vi "Ball Intake System.vi"(10 "Outtake":bool, 11 "Intake":bool) -> ()   [LabVIEW 2018]
panel:
  in  "Scaling factor":dbl=0.5
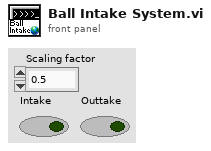
[diagram p1: front panel]
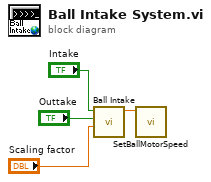
[diagram p0: block diagram]
diagram:
  n1 = call "Ball Intake.vi"("Scaling factor"="Scaling factor", "Outtake"="Outtake", "Intake"="Intake") -> ("IntakeSpeed"=w4:dbl)  [unwired: 8 in]
  n2 = call "SetBallMotorSpeed.vi"("IntakeSpeed"=w4) -> ()  [unwired: 11 in]
